vi "ComputeNumberofPoints.vi"(10 "Window, cm":dbl=42.0, 11 "Nyquist, mm":dbl=28.0) -> (1 "Window adjusted, cm":dbl, 2 "Total points":dbl, 3 "Points per side":dbl)   [LabVIEW 2019]
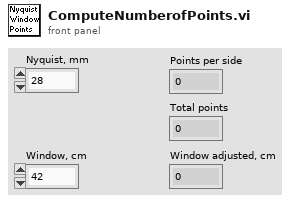
[diagram p1: front panel]
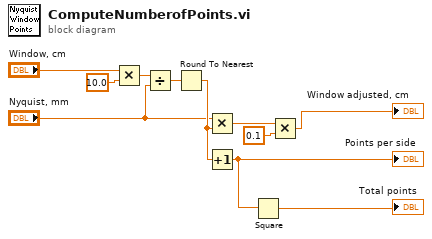
[diagram p0: block diagram]
diagram:
  n1 = Multiply(x="Window, cm", y=10.0) -> (x*y=w9:dbl)
  n2 = Divide(x=w9, y="Nyquist, mm") -> (x/y=w8:dbl)
  n3 = Round To Nearest(number=w8) -> (nearest integer value=w5:dbl)
  n4 = Multiply(x="Nyquist, mm", y=w5) -> (x*y=w3:dbl)
  n5 = Increment(x=w5) -> (x+1=w7:dbl)
  "Points per side" <- w7
  n6 = Square(x=w7) -> (x^2=→"Total points":dbl)
  n7 = Multiply(x=w3, y=0.1) -> (x*y=→"Window adjusted, cm":dbl)
